vi "rql_EHL Clear Filter - Value Change.vi"(4 "Show in Debugger?":bool=TRUE, 6 "Message Priority":T1=enum."Normal", 8 "error in":errorcluster, 9 "Data in":T2, 11 "Message Log in":refnum<class "Message Log.lvclass">) -> (0 "error out":errorcluster, 3 "dup Message Log out":refnum<class "Message Log.lvclass">)   [LabVIEW 2017, in "Message Log.lvclass"]
doc: "This VI sends a <b>Local API Request</b> message to an MHL case of the Worker that owns this VI.\n---\nDelete all elements in the fitler element cluster, and update the UI Message Log with all elements."
uses:
  Message Log.lvclass
  C:/Program Files (x86)/National Instruments/LabVIEW 2017/vi.lib/addons/_Workers/Library/Classes/Worker/Worker.lvclass
  rql_EHL Clear Filter - Value Change.ctl
  <vilib>/addons/_Workers/Library/Classes/Message/Priority.ctl
  <vilib>/addons/_Workers/Library/Classes/Worker/Worker.lvclass/Worker.ctl
  <vilib>/addons/_Workers/Library/Classes/Worker/Worker.lvclass
  <vilib>/addons/_Workers/Library/Classes/Message/Message.lvclass
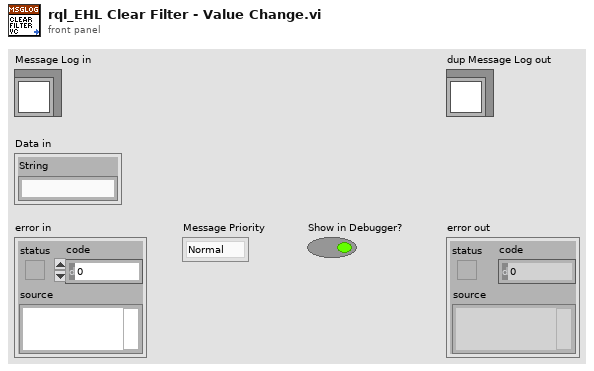
[diagram p1: front panel]
types:
  T1 = typedef "Workers.lvlib/Message.lvclass/Priority.ctl" = enum16{"Low", "Normal", "High"}
  T2 = typedef "Message Log.lvclass/rql_EHL Clear Filter - Value Change.ctl" = cluster{"String":string}
  T3 = typedef "Workers.lvlib/Case Label.ctl" = string
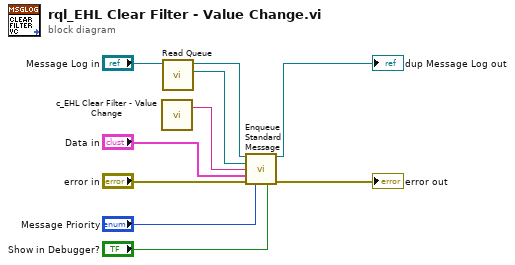
[diagram p0: block diagram]
diagram:
  n1 = call "c_EHL Clear Filter - Value Change.vi"() -> ("Case Label"=w4:T3)  [unwired: 1 in]
  n2 = call <vilib>:"Read Queue.vi"("Worker_"="Message Log in") -> ("Message Queue out"=w5:refnum<class "Message Queue.lvclass">, "dup Worker_out"=w6:refnum<class "Message Log.lvclass">)  [unwired: 9 in]
  n3 = call-dynamic "Enqueue Standard Message.vi"("Worker"=w6, "Message Queue"=w5, "Case Label"=w4, "Data"="Data in", "error in (no error)"="error in", "Priority (Normal)"="Message Priority", "Send Message to Debugger? (T)"="Show in Debugger?") -> ("dup Worker out"=→"dup Message Log out":refnum<class "Message Log.lvclass">, "error out"=→"error out":errorcluster)  [unwired: 7 in]
